vi "BIO_new_ssl_connect.vi"(8 "error in (no error)":errorcluster, 11 "SSL-Context in":refnum<class "SSL-Context.lvclass">) -> (0 "error out":errorcluster, 2 "BIO out":refnum<class "BIO.lvclass">, 3 "SSL-Context out":refnum<class "SSL-Context.lvclass">)   [LabVIEW 2013, in "SSL_Lib.lvlib" / "SSL-Context.lvclass"]
uses:
  SSL-Context.lvclass
  BIO/BIO.lvclass
  SSL-Lib/SSL-Lib.lvclass/SSL-Lib.ctl
  SSL-Context.lvclass/SSL-Context.ctl
  BIO/BIO.lvclass/BIO.ctl
  SSL-Lib/Read SSL Library Path.vi
  Read Handle.vi
  BIO/Write Handle.vi
  SSL-Lib/SSL-Lib.lvclass
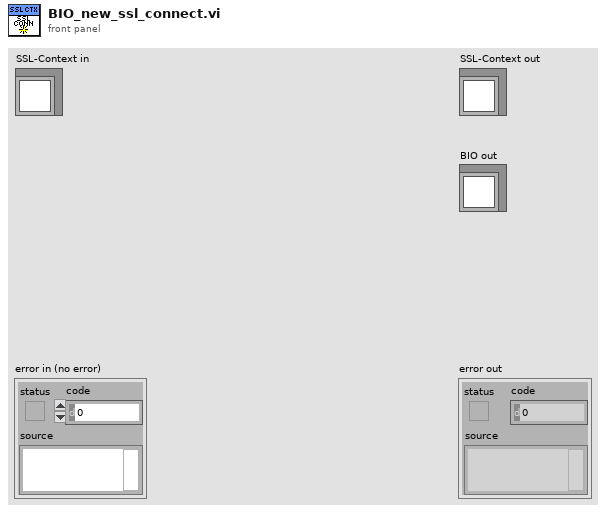
[diagram p1: front panel]
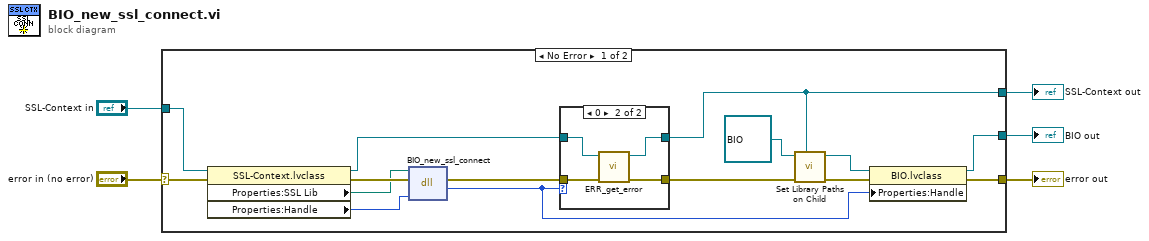
[diagram p0: block diagram]
diagram:
  n1 = case shown="No Error" "error in (no error)" {
    selector: "error in (no error)" -> [w20 w28]
    tunnel: [w12 w28] -> w4
    tunnel: [w8 w27] -> w2
    tunnel: "SSL-Context in" -> [w18 w27]
    tunnel: [w11 _] -> w1
    frame No Error {
      n2 = property class="SSL-Context.lvclass"(reference=w18, error in=w20) -> (reference out=w9:refnum<class "SSL-Context.lvclass">, error out=w19:errorcluster, "Properties:SSL Lib"=w17:path, "Properties:Handle"=w16:u64)
      n3 = dll-call lib="C:/Program Files (x86)/National Instruments/Shared/nissl/NIssleay32.dll" fn="BIO_new_ssl_connect"(path in=w17, error in=w19, "SSL_CTX"=w16) -> (error out=w10:errorcluster, "return type"=w6:u64)  [unwired: 2 in, 1 out]
      n4 = case shown="0" w6 {
        tunnel: w10 -> [w22 w26]
        tunnel: w9 -> [w21 w25]
        tunnel: [w21 w24] -> w8
        tunnel: [w22 w23] -> w7
        frame Default {
        }
        frame 0 {
          n5 = call "ERR_get_error.vi"("error in (no error)"=w26, "SSL-Lib in"=w25) -> ("error out"=w23:errorcluster, "SSL-Lib out"=w24:refnum<class "SSL-Context.lvclass">)  [unwired: 8 in]
        }
      }
      n6 = call-dynamic "Set Library Paths on Child.vi"(7:"SSL-Lib in"=w8, "error in (no error)"=w7, 11:"SSL-Lib in"=refnum<class "BIO.lvclass"> refnum ("SSL_Lib.lvlib:BIO.lvclass")) -> ("error out"=w14:errorcluster, "SSL-Lib out"=w13:refnum<class "BIO.lvclass">)  [unwired: 7 in]
      n7 = property class="BIO.lvclass"(reference=w13, error in=w14, "Properties:Handle"=w6) -> (reference out=w11:refnum<class "BIO.lvclass">, error out=w12:errorcluster)
    }
    frame Error {
    }
  }
  "error out" <- w4
  "SSL-Context out" <- w2
  "BIO out" <- w1
